vi "Auto_Routine_Balance.vi"(8 "error in (no error)":errorcluster) -> (0 "error out":errorcluster)   [LabVIEW 2020]
doc: "Balances\n\ninputs:\n--ErrorIn--\n\noutputs:\n--ErrorOut--"
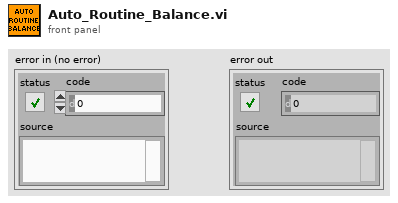
[diagram p1: front panel]
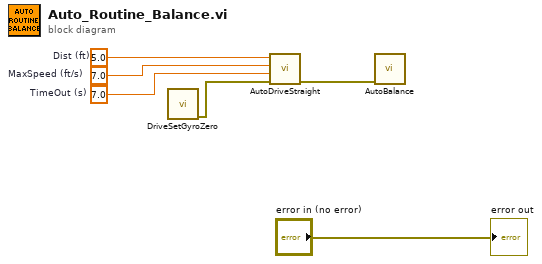
[diagram p0: block diagram]
diagram:
  w3 = 7.0  # TimeOut (s)
  w4 = 7.0  # MaxSpeed (ft/s)
  w2 = 5.0  # Dist (ft)
  n1 = call "DriveSetGyroZero.vi"() -> ("error out"=w6:errorcluster)  [unwired: 11 in]
  n2 = call "AutoDriveStraight.vi"("error in (no error)"=w6, "TimeOut (s)"=w3, "MaxSpeed (ft/s)"=w4, "Dist (ft)"=w2) -> ("error out"=w5:errorcluster)  [unwired: 7 in]
  n3 = call "AutoBalance.vi"("error in (no error)"=w5) -> ()  [unwired: 10 in, 1 out]
  "error out" <- "error in (no error)"
